vi "SeqLoop.vi"(6 "SEQ STEP Display":refnum<notifier>, 8 "error in (no error)":errorcluster, 9 "SEQ":refnum<queue>, 10 "CORE":refnum<queue>, 11 "WINFAS 2 Data Queue":T3) -> (0 "error out":errorcluster)   [LabVIEW 2014, in "SeqLoop.lvlib"]
uses:
  SeqLoop.lvlib
  APIs/Message Queue/Message Cluster.ctl
  APIs/Data Queue/All Data Queues Cluster.ctl
  APIs/Data Queue/Acquisition Data 1 Sample Cluster.ctl
  APIs/Data Queue/Control Data Cluster.ctl
  APIs/Data Queue/Async Acquisition Data Cluster.ctl
  TypeDefs/STEP Display.ctl
  Mimico Display/TypeDefs/Mimic Data.ctl
  Mimico Display/TypeDefs/BG Image.ctl
  Mimico Display/TypeDefs/mObject.ctl
  TypeDefs/Sequence.ctl
  Classes/STEP/STEP.lvclass
  TypeDefs/LogicParsedExpression.ctl
  TypeDefs/Program.ctl
  TypeDefs/HW InOut MAP.ctl
  TypeDefs/Variables State.ctl
  TypeDefs/STEP State.ctl
  Classes/Measurement/Measurement.lvclass
  Classes/AutoZero/AutoZero.lvclass
  Classes/Measurement wRelev/Measurement wRelev.lvclass
  Classes/Relev/Relev.lvclass
  Classes/Measurement wMaster/Measurement wMaster.lvclass
  Classes/Mastering/Mastering.lvclass
  Classes/Scale Calibration/Scale Calibration.lvclass
  APIs/Message Queue/Enqueue Message (Single).vi
  SEQ Monitoring Global Variables.vi
  APIs/Message Queue/WINFAS 2 Message Queue.lvlib
  APIs/Data Queue/WINFAS 2 Data Queue.lvlib
  Mimico Display/Mimico Display.lvlib
panel:
  in  "Empty Sequence":T1
  in  "Current Sequence":T1
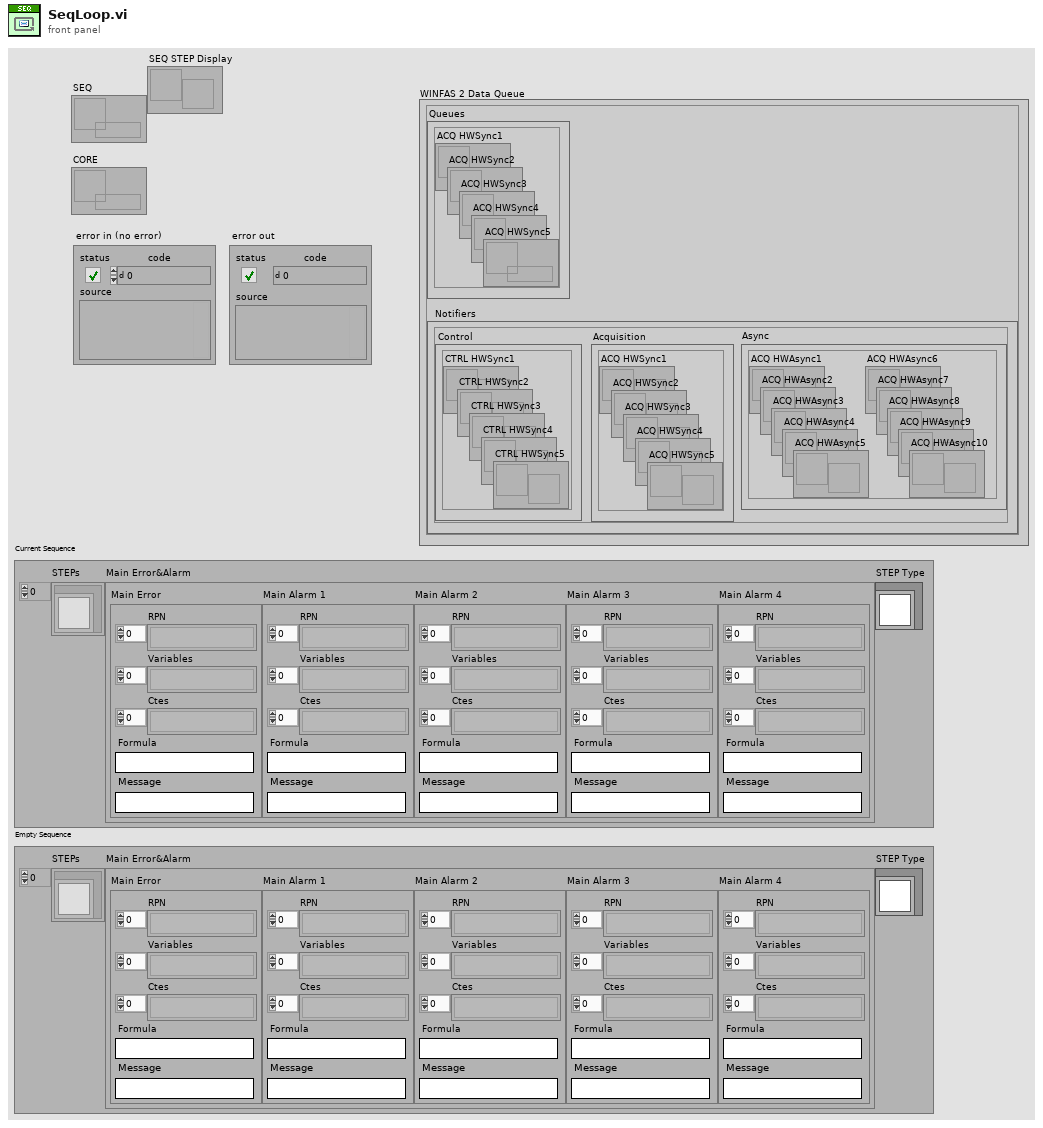
[diagram p1: front panel]
types:
  T1 = typedef "SeqLoop.lvlib/Sequence.ctl" = cluster{"STEPs":refnum<class "STEP.lvclass">[], "Main Error&Alarm":cluster{"Main Error":T2, "Main Alarm 1":T2, "Main Alarm 2":T2, "Main Alarm 3":T2, "Main Alarm 4":T2}, "STEP Type":refnum<class "STEP.lvclass">}
  T2 = typedef "SeqLoop.lvlib/LogicParsedExpression.ctl" = cluster{"RPN ":string[], "Variables":string[], "Ctes":string[], "Formula":string, "Message":string}
  T3 = typedef "WINFAS 2 Data Queue.lvlib/All Data Queues Cluster.ctl" = cluster{"Queues":cluster{"ACQ HWSync1":refnum<queue>, "ACQ HWSync2":refnum<queue>, "ACQ HWSync3":refnum<queue>, "ACQ HWSync4":refnum<queue>, "ACQ HWSync5":refnum<queue>}, "Notifiers":cluster{"Control":cluster{"CTRL HWSync1":refnum<notifier>, "CTRL HWSync2":refnum<notifier>, "CTRL HWSync3":refnum<notifier>, "CTRL HWSync4":refnum<notifier>, "CTRL HWSync5":refnum<notifier>}, "Acquisition":cluster{"ACQ HWSync1":refnum<notifier>, "ACQ HWSync2":refnum<notifier>, "ACQ HWSync3":refnum<notifier>, "ACQ HWSync4":refnum<notifier>, "ACQ HWSync5":refnum<notifier>}, "Async":cluster{"ACQ HWAsync1":refnum<notifier>, "ACQ HWAsync2":refnum<notifier>, "ACQ HWAsync3":refnum<notifier>, "ACQ HWAsync4":refnum<notifier>, "ACQ HWAsync5":refnum<notifier>, "ACQ HWAsync6":refnum<notifier>, "ACQ HWAsync7":refnum<notifier>, "ACQ HWAsync8":refnum<notifier>, "ACQ HWAsync9":refnum<notifier>, "ACQ HWAsync10":refnum<notifier>}}}
  T4 = typedef "SeqLoop.lvlib/STEP State.ctl" = enum16{"Stopped", "First Call", "Idle...", "Advance OK", "Alarm", "Output Security", "Error"}
  T5 = typedef "SeqLoop.lvlib/Variables State.ctl" = cluster{"I":bool[], "P":bool[], "N":bool[], "T":bool[], "X":bool[], "Timer":u32[], "Wait":u32, "Wait?":bool, "Jump":cluster{"Jumping?":bool, "Previous STEP to Jump":u32, "Initial Jump STEP":u32, "STEP Count":u32, "Loop Count":u32, "Number of STEPs":u32, "Repetitions":u32}, "Reset?":bool}
  T6 = typedef "SeqLoop.lvlib/HW InOut MAP.ctl" = cluster{"Inputs":cluster{"Entrada":i32, "Descripción":string, "Habilitada?":bool}[][], "Outputs":cluster{"Salida":i32, "Descripción":string, "Habilitada?":bool, "Formula":string, "Tipo de Salida":string}[][]}
  T7 = typedef "SeqLoop.lvlib/Program.ctl" = cluster{"Prog. Data":cluster{"Tipo de Programa":string, "Operación":i32, "Pieza":i32, "Descripción":string, "Nombre Programa":string, "Autor":string, "Cód. Prog.":i32, "Diseño":string, "Total Meds.:":i32, "Total Meds. Aux.:":i32}, "All Sequences":cluster{"Measurement":T1, "AutoZero":T1, "Special":T1}}
  T8 = cluster{"CTRL HWSync1":refnum<notifier>, "CTRL HWSync2":refnum<notifier>, "CTRL HWSync3":refnum<notifier>, "CTRL HWSync4":refnum<notifier>, "CTRL HWSync5":refnum<notifier>}
  T9 = cluster{"File Direction":path, "Progs Data":variant}
  T10 = cluster{"element":cluster{"File Direction":path, "Progs Data":variant}, "Program Type":string}
  T11 = typedef "SeqLoop.lvlib/HW CTRL Data.ctl" = cluster{"Inputs":bool[], "Encoder 1":sgl, "Encoder 2":sgl, "Encoder 3":sgl, "Encoder 4":sgl, "Encoder 5":sgl}
  T12 = cluster{"Alarm 1":bool, "Alarm 2":bool, "Alarm 3":bool, "Alarm 4":bool, "Main Err&Alarm?":bool}
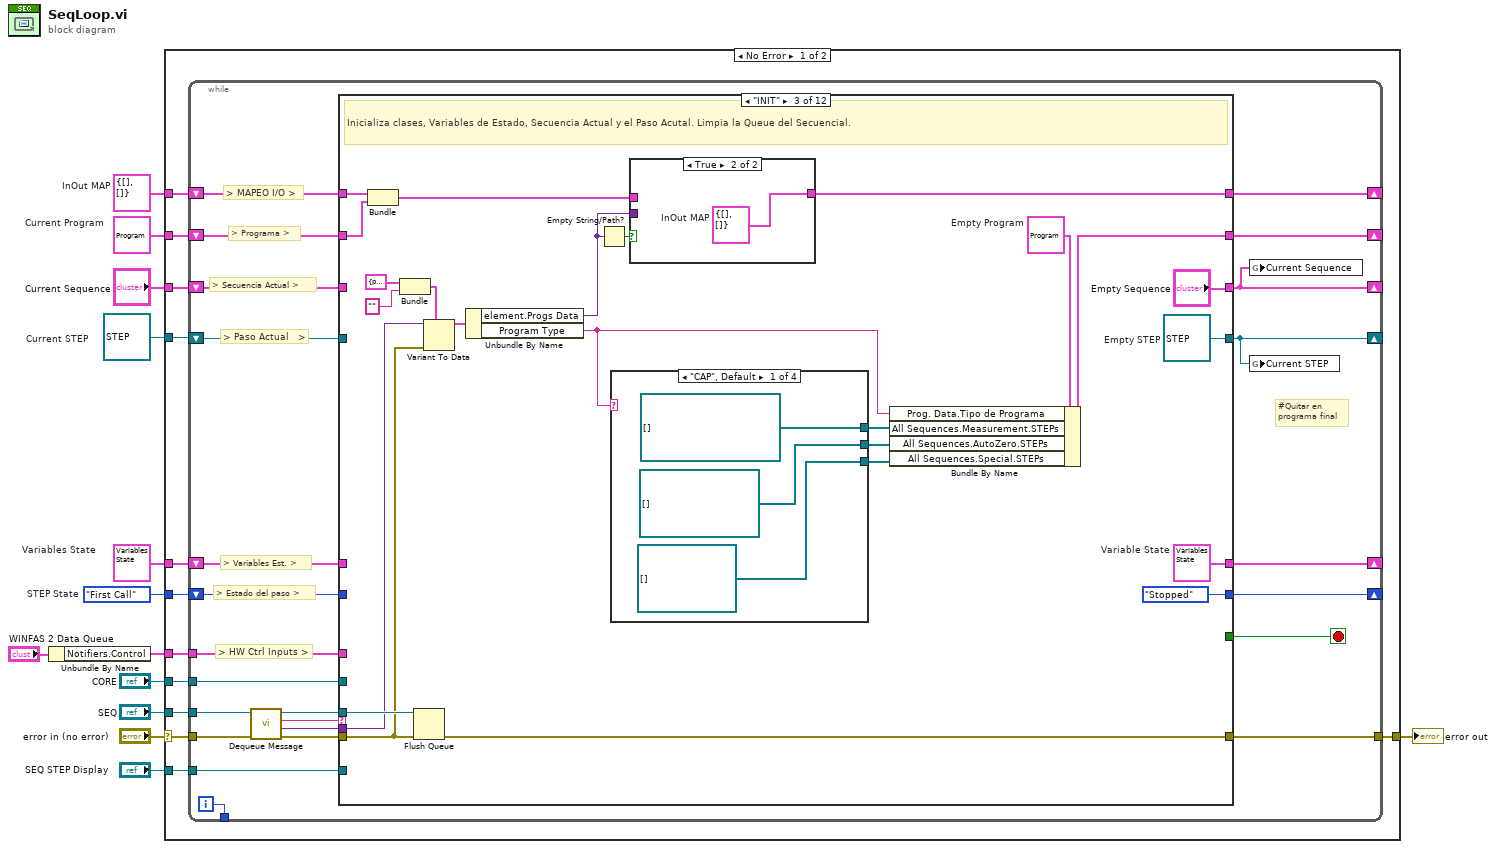
[diagram p0: block diagram]
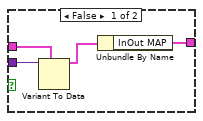
[diagram p4: hidden frame]
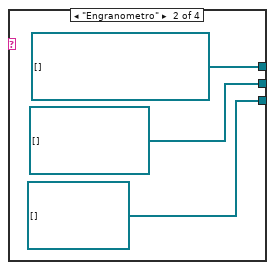
[diagram p5: hidden frame]
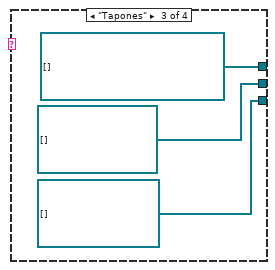
[diagram p6: hidden frame]
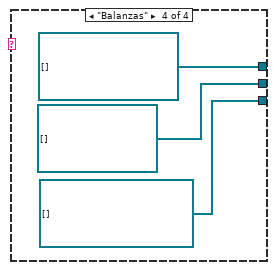
[diagram p7: hidden frame]
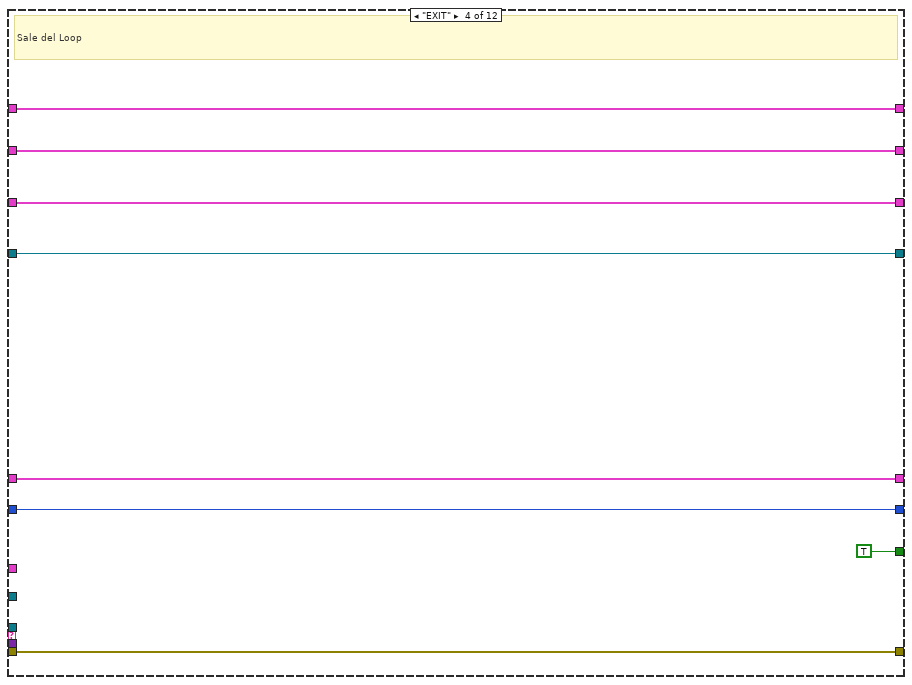
[diagram p8: hidden frame]
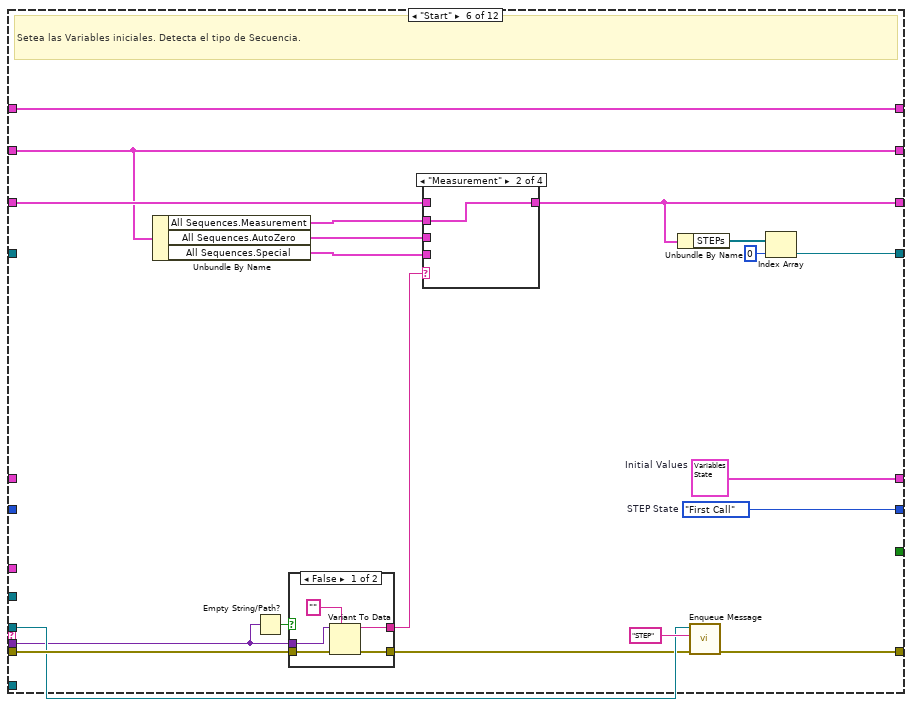
[diagram p10: hidden frame]
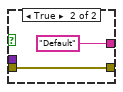
[diagram p11: hidden frame]
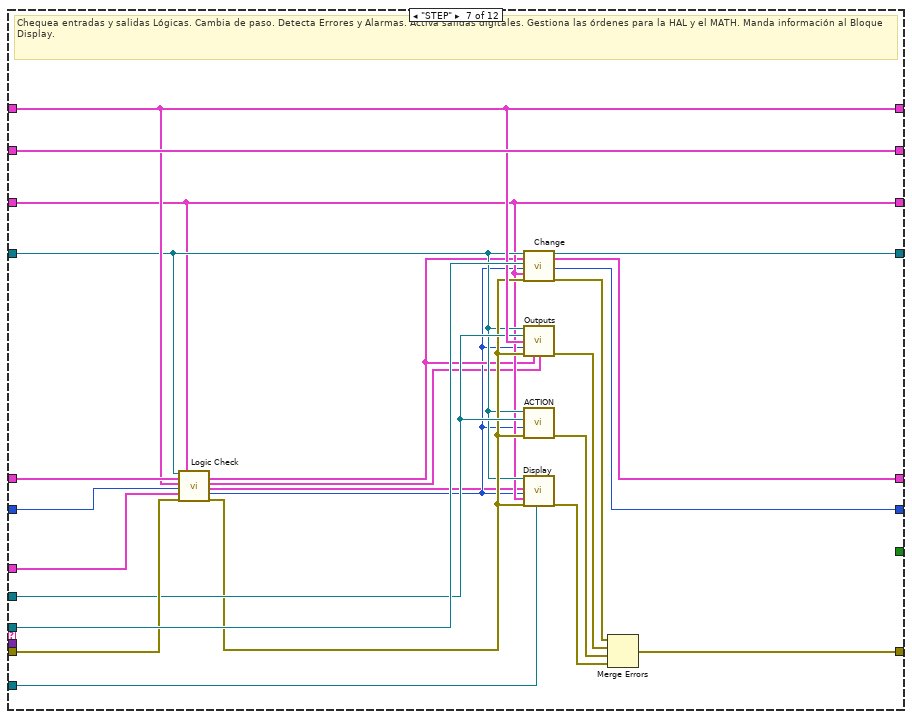
[diagram p15: hidden frame]
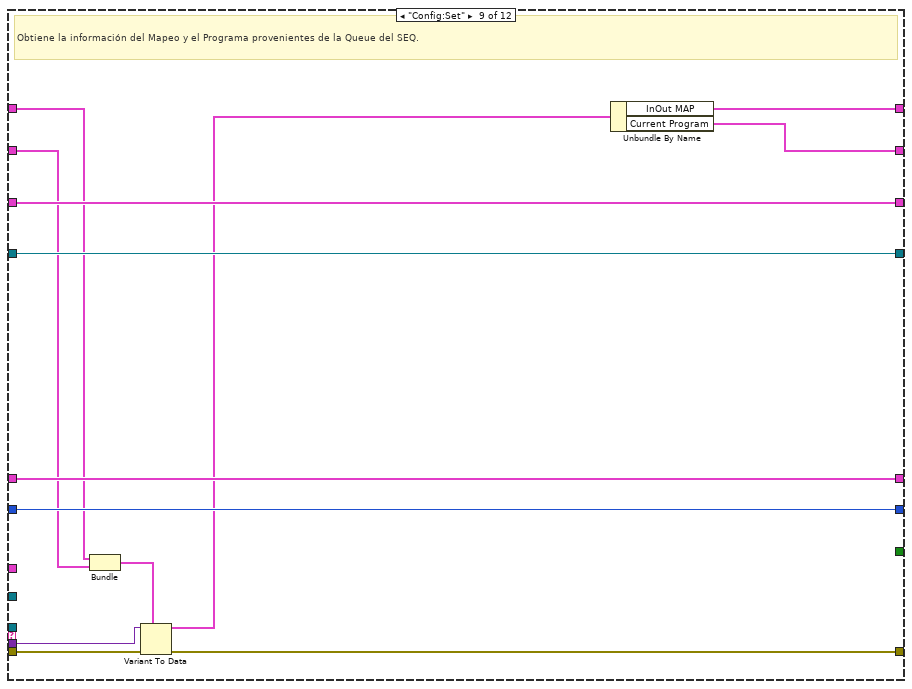
[diagram p17: hidden frame]
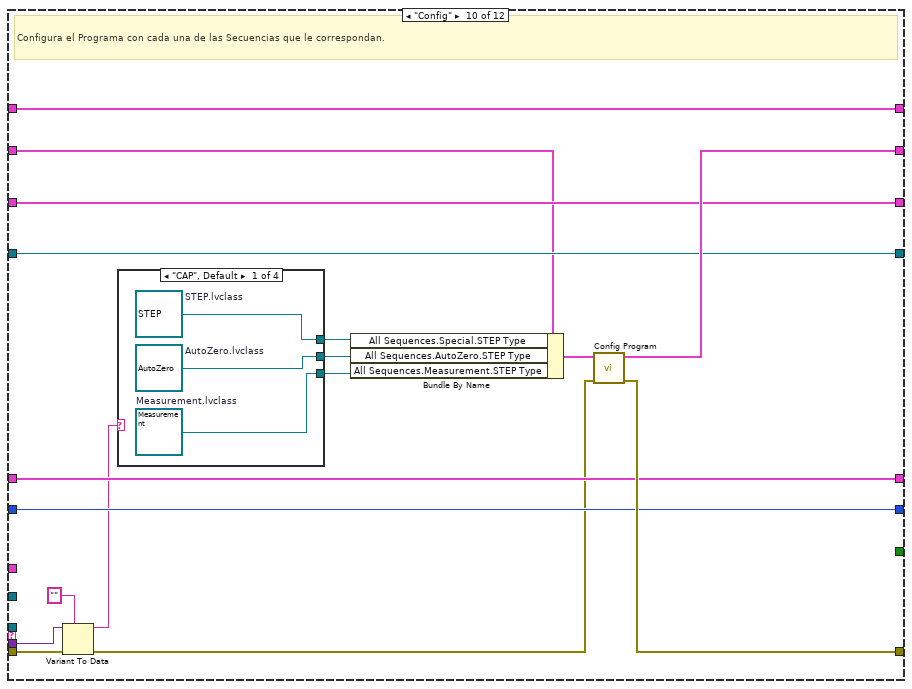
[diagram p18: hidden frame]
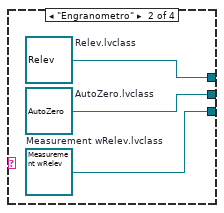
[diagram p19: hidden frame]
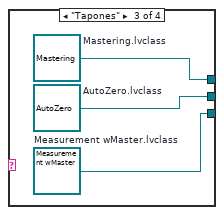
[diagram p20: hidden frame]
diagram:
  w3 = refnum<class "STEP.lvclass"> refnum  # Current STEP
  w6 = STEP_State."First Call"  # STEP State
  w7 = T5 {"I"=[], "P"=[], "N"=[], "T"=[], "X"=[], "Timer"=[], "Wait"=0, "Wait?"=FALSE, "Jump"={"Jumping?"=FALSE, "Previous STEP to Jump"=0, "Initial Jump STEP"=0, "STEP Count"=0, "Loop Count"=0, "Number of STEPs"=0, "Repetitions"=0}, "Reset?"=FALSE}  # Variables State
  w9 = T6 {"Inputs"=[], "Outputs"=[]}  # InOut MAP
  w8 = T7 {"Prog. Data"={"Tipo de Programa"="", "Operación"=0, "Pieza"=0, "Descripción"="", "Nombre Programa"="", "Autor"="", "Cód. Prog."=0, "Diseño"="", "Total Meds.:"=0, "Total Meds. Aux.:"=0}, "All Sequences"={"Measurement"={"STEPs"=[], "Main Error&Alarm"={"Main Error"={"RPN "=[], "Variables"=[], "Ctes"=[], "Formula"="", "Message"=""}, "Main Alarm 1"={"RPN "=[], "Variables"=[], "Ctes"=[], "Formula"="", "Message"=""}, "Main Alarm 2"={"RPN "=[], "Variables"=[], "Ctes"=[], "Formula"="", "Message"=""}, "Main Alarm 3"={"RPN "=[], "Variables"=[], "Ctes"=[], "Formula"="", "Message"=""}, "Main Alarm 4"={"RPN "=[], "Variables"=[], "Ctes"=[], "Formula"="", "Message"=""}}, "STEP Type"=refnum}, "AutoZero"={"STEPs"=[], "Main Error&Alarm"={"Main Error"={"RPN "=[], "Variables"=[], "Ctes"=[], "Formula"="", "Message"=""}, "Main Alarm 1"={"RPN "=[], "Variables"=[], "Ctes"=[], "Formula"="", "Message"=""}, "Main Alarm 2"={"RPN "=[], "Variables"=[], "Ctes"=[], "Formula"="", "Message"=""}, "Main Alarm 3"={"RPN "=[], "Variables"=[], "Ctes"=[], "Formula"="", "Message"=""}, "Main Alarm 4"={"RPN "=[], "Variables"=[], "Ctes"=[], "Formula"="", "Message"=""}}, "STEP Type"=refnum}, "Special"={"STEPs"=[], "Main Error&Alarm"={"Main Error"={"RPN "=[], "Variables"=[], "Ctes"=[], "Formula"="", "Message"=""}, "Main Alarm 1"={"RPN "=[], "Variables"=[], "Ctes"=[], "Formula"="", "Message"=""}, "Main Alarm 2"={"RPN "=[], "Variables"=[], "Ctes"=[], "Formula"="", "Message"=""}, "Main Alarm 3"={"RPN "=[], "Variables"=[], "Ctes"=[], "Formula"="", "Message"=""}, "Main Alarm 4"={"RPN "=[], "Variables"=[], "Ctes"=[], "Formula"="", "Message"=""}}, "STEP Type"=refnum}}}  # Current Program
  n1 = Unbundle By Name("WINFAS 2 Data Queue") -> ("Notifiers.Control"=w4:T8)
  n2 = case shown="No Error" "error in (no error)" {
    selector: "error in (no error)" -> [w25 w245]
    tunnel: [w18 w245] -> w12
    tunnel: "CORE" -> [w24 _]
    tunnel: "SEQ" -> [w23 _]
    tunnel: w9 -> [w22 _]
    tunnel: w8 -> [w21 _]
    tunnel: "Current Sequence" -> [w17 _]
    tunnel: w7 -> [w20 _]
    tunnel: "SEQ STEP Display" -> [w19 _]
    tunnel: w6 -> [w16 _]
    tunnel: w4 -> [w15 _]
    tunnel: w3 -> [w14 _]
    frame No Error {
      n3 = while {
        tunnel: w25 -> [w45]
        tunnel: [w33] -> w18
        tunnel: w23 -> [w46]
        shift-right: [w47] -> _
        shift-left: w20 -> [w48]
        shift-right: [w40] -> _
        shift-left: w22 -> [w41]
        shift-right: [w38] -> _
        shift-left: w21 -> [w39]
        tunnel: w24 -> [w37]
        tunnel: w19 -> [w36]
        shift-right: [w27] -> _
        shift-left: w17 -> [w34]
        tunnel: w15 -> [w35]
        shift-right: [w28] -> _
        shift-left: w14 -> [w30]
        shift-right: [w29] -> _
        shift-left: w16 -> [w31]
        tunnel: [w26] -> _
        i -> [w26]
        stop <- w49 stop-if-true
        # "#Quitar en\nprograma final"
        # "> HW Ctrl Inputs >"
        # "> Variables Est. >"
        # "> Estado del paso >"
        # "> Paso Actual   >"
        # "> Secuencia Actual >"
        # "> Programa >"
        # "> MAPEO I/O >"
        n4 = call "Dequeue Message.vi"("error in (no error)"=w45, "Message Queue"=w46) -> ("error out"=w44:errorcluster, "Message Data"=w42:variant, "Message"=w43:string, "dup Message Queue"=w32:refnum<queue>)  [unwired: 6 in]
        n5 = case shown="\"INIT\"" w43 {
          tunnel: [w55 w59 w85 w110 w119 w131 w168 w180 w183 w211 w232 w241] -> w33
          tunnel: w44 -> [w55 w59 w80 w110 w119 w137 w163 w180 w193 w202 w224 w242]
          tunnel: w42 -> [_ _ w79 _ _ w121 _ _ w192 w195 _ _]
          tunnel: [_ _ _ TRUE _ _ _ _ _ _ _ _] -> w49
          tunnel: w48 -> [w56 w63 _ w111 w118 _ w166 w181 w194 w210 w231 w244]
          tunnel: [w56 w63 w86 w111 w118 w128 w156 w181 w194 w210 w231 w244] -> w47
          tunnel: w41 -> [w52 w61 w69 w107 w116 w135 w162 w177 w186 w209 w230 w235]
          tunnel: [w52 w61 w67 w107 w116 w135 w162 w177 w189 w209 w229 w235] -> w40
          tunnel: w39 -> [w54 w62 w68 w109 w117 w132 w171 w179 w185 w200 w228 w234]
          tunnel: [w54 w62 w81 w109 w117 w132 w171 w179 w190 w208 w228 w234] -> w38
          tunnel: w37 -> [_ _ _ _ _ _ w161 _ _ _ _ w243]
          tunnel: w36 -> [_ _ _ _ _ _ w165 _ _ _ _ _]
          tunnel: [w53 w60 "Empty Sequence" w108 w115 w124 w155 w178 w191 w207 w227 w239] -> w27
          tunnel: w34 -> [w53 w60 _ w108 w115 w133 w155 w178 w191 w207 w227 w239]
          tunnel: w35 -> [_ _ _ _ _ _ w167 _ _ _ _ _]
          tunnel: w32 -> [_ _ w87 _ _ w134 w169 _ _ _ _ _]
          tunnel: w31 -> [w50 w57 _ w105 w113 _ w164 w175 w187 w205 w225 w237]
          tunnel: [w51 w58 w84 w106 w114 w122 w172 w176 w188 w206 w226 w238] -> w28
          tunnel: w30 -> [w51 w58 _ w106 w114 _ w157 w176 w188 w206 w226 w238]
          tunnel: [w50 w57 STEP_State."Stopped" ("STEP State") w105 w113 w126 w170 w175 w187 w205 w225 w237] -> w29
          frame "----LOOP----" {
            # "Bloque que adminte futuras configuraciones al inicio."
          }
          frame Default {
          }
          frame "INIT" {
            w84 = refnum<class "STEP.lvclass"> refnum  # Empty STEP
            w82 = T7 {"Prog. Data"={"Tipo de Programa"="", "Operación"=0, "Pieza"=0, "Descripción"="", "Nombre Programa"="", "Autor"="", "Cód. Prog."=0, "Diseño"="", "Total Meds.:"=0, "Total Meds. Aux.:"=0}, "All Sequences"={"Measurement"={"STEPs"=[], "Main Error&Alarm"={"Main Error"={"RPN "=[], "Variables"=[], "Ctes"=[], "Formula"="", "Message"=""}, "Main Alarm 1"={"RPN "=[], "Variables"=[], "Ctes"=[], "Formula"="", "Message"=""}, "Main Alarm 2"={"RPN "=[], "Variables"=[], "Ctes"=[], "Formula"="", "Message"=""}, "Main Alarm 3"={"RPN "=[], "Variables"=[], "Ctes"=[], "Formula"="", "Message"=""}, "Main Alarm 4"={"RPN "=[], "Variables"=[], "Ctes"=[], "Formula"="", "Message"=""}}, "STEP Type"=refnum}, "AutoZero"={"STEPs"=[], "Main Error&Alarm"={"Main Error"={"RPN "=[], "Variables"=[], "Ctes"=[], "Formula"="", "Message"=""}, "Main Alarm 1"={"RPN "=[], "Variables"=[], "Ctes"=[], "Formula"="", "Message"=""}, "Main Alarm 2"={"RPN "=[], "Variables"=[], "Ctes"=[], "Formula"="", "Message"=""}, "Main Alarm 3"={"RPN "=[], "Variables"=[], "Ctes"=[], "Formula"="", "Message"=""}, "Main Alarm 4"={"RPN "=[], "Variables"=[], "Ctes"=[], "Formula"="", "Message"=""}}, "STEP Type"=refnum}, "Special"={"STEPs"=[], "Main Error&Alarm"={"Main Error"={"RPN "=[], "Variables"=[], "Ctes"=[], "Formula"="", "Message"=""}, "Main Alarm 1"={"RPN "=[], "Variables"=[], "Ctes"=[], "Formula"="", "Message"=""}, "Main Alarm 2"={"RPN "=[], "Variables"=[], "Ctes"=[], "Formula"="", "Message"=""}, "Main Alarm 3"={"RPN "=[], "Variables"=[], "Ctes"=[], "Formula"="", "Message"=""}, "Main Alarm 4"={"RPN "=[], "Variables"=[], "Ctes"=[], "Formula"="", "Message"=""}}, "STEP Type"=refnum}}}  # Empty Program
            w86 = T5 {"I"=[], "P"=[], "N"=[], "T"=[], "X"=[], "Timer"=[], "Wait"=0, "Wait?"=FALSE, "Jump"={"Jumping?"=FALSE, "Previous STEP to Jump"=0, "Initial Jump STEP"=0, "STEP Count"=0, "Loop Count"=0, "Number of STEPs"=0, "Repetitions"=0}, "Reset?"=FALSE}  # Variable State
            # "Inicializa clases, Variables de Estado, Secuencia Actual y el Paso Acutal. Limpia la Queue del Secuencial."
            n6 = Bundle("InOut MAP"=w69, "Current Program"=w68) -> (w70:cluster{"InOut MAP":T6, "Current Program":T7})  [unwired: 1 in]
            n7 = Bundle("element"=T9 {"File Direction"=path "", "Progs Data"=variant}, "Program Type"="") -> (w71:T10)  [unwired: 1 in]
            n8 = Flush Queue(queue=w87, error in (no error)=w80) -> (error out=w85:errorcluster)  [unwired: 2 out]
            n9 = Variant To Data(error in=w80, type=w71, Variant=w79) -> (data=w74:T10)  [unwired: 1 out]
            n10 = Unbundle By Name(w74) -> ("element.Progs Data"=w66:variant, "Program Type"=w64:string)
            n11 = Empty String/Path?(string/path=w66) -> (empty?=w65:bool)
            n12 = case shown="\"CAP\", Default" w64 {
              tunnel: [refnum<class "Measurement.lvclass">[] [] refnum<class "Measurement wRelev.lvclass">[] [] refnum<class "Measurement wMaster.lvclass">[] [] refnum<class "Measurement.lvclass">[] []] -> w78
              tunnel: [refnum<class "AutoZero.lvclass">[] [] refnum<class "AutoZero.lvclass">[] [] refnum<class "AutoZero.lvclass">[] [] refnum<class "AutoZero.lvclass">[] []] -> w77
              tunnel: [refnum<class "STEP.lvclass">[] [] refnum<class "Relev.lvclass">[] [] refnum<class "Mastering.lvclass">[] [] refnum<class "Scale Calibration.lvclass">[] []] -> w76
              frame "CAP", Default {
              }
              frame "Engranometro" {
              }
              frame "Tapones" {
              }
              frame "Balanzas" {
              }
            }
            n13 = case shown="True" w65 {
              tunnel: w70 -> [w91 _]
              tunnel: [w89 w92] -> w67
              tunnel: w66 -> [w88 _]
              frame False {
                n14 = Variant To Data(type=w91, Variant=w88) -> (data=w90:cluster{"InOut MAP":T6, "Current Program":T7})  [unwired: 1 in, 1 out]
                n15 = Unbundle By Name(w90) -> ("InOut MAP"=w89:T6)
              }
              frame True {
                w92 = T6 {"Inputs"=[], "Outputs"=[]}  # InOut MAP
              }
            }
            n16 = Bundle By Name(cluster=w82, "Prog. Data.Tipo de Programa"=w64, "All Sequences.Measurement.STEPs"=w78, "All Sequences.AutoZero.STEPs"=w77, "All Sequences.Special.STEPs"=w76) -> (w81:T7)
          }
          frame "EXIT" {
            # "Sale del Loop"
          }
          frame "----ACTION----" {
          }
          frame "Start" {
            w126 = STEP_State."First Call"  # STEP State
            w128 = T5 {"I"=[], "P"=[], "N"=[], "T"=[], "X"=[], "Timer"=[], "Wait"=0, "Wait?"=FALSE, "Jump"={"Jumping?"=FALSE, "Previous STEP to Jump"=0, "Initial Jump STEP"=0, "STEP Count"=0, "Loop Count"=0, "Number of STEPs"=0, "Repetitions"=0}, "Reset?"=FALSE}  # Initial Values
            # "Setea las Variables iniciales. Detecta el tipo de Secuencia."
            n17 = Unbundle By Name(w132) -> ("All Sequences.Measurement"=w139:T1, "All Sequences.AutoZero"=w138:T1, "All Sequences.Special"=w129:T1)
            n18 = Empty String/Path?(string/path=w121) -> (empty?=w120:bool)
            n19 = case shown="False" w120 {
              tunnel: w137 -> [w144 w146]
              tunnel: [w142 "Default"] -> w130
              tunnel: [w141 w146] -> w125
              tunnel: w121 -> [w140 _]
              frame False {
                n20 = Variant To Data(error in=w144, type="", Variant=w140) -> (data=w142:string, error out=w141:errorcluster)
              }
              frame True {
              }
            }
            n21 = case shown="\"Measurement\"" w130 {
              tunnel: w139 -> [_ w148 _ _]
              tunnel: w138 -> [_ _ w149 _]
              tunnel: [w147 w148 w149 w150] -> w124
              tunnel: w133 -> [w147 _ _ _]
              tunnel: w129 -> [_ _ _ w150]
              frame Default {
              }
              frame "Measurement" {
              }
              frame "Auto-Zero" {
              }
              frame "Special" {
              }
            }
            n22 = Unbundle By Name(w124) -> ("STEPs"=w123:refnum<class "STEP.lvclass">[])
            n23 = call-poly "Enqueue Message.vi"("error in (no error)"=w125, "Message"="STEP", "Message Queue"=w134) -> ("error out"=w131:errorcluster)  [unwired: 7 in, 1 out]
            n24 = Index Array(array=w123, index=0) -> (element=w122:refnum<class "STEP.lvclass">)
          }
          frame "STEP" {
            # "Chequea entradas y salidas Lógicas. Cambia de paso. Detecta Errores y Alarmas. Activa salidas digitales. Gestiona las órdenes para la HAL y el MATH. Manda información al Bloque Display."
            n25 = call "Logic Check.vi"("STEP in"=w157, "Variables State in"=w166, "HW InOut MAP"=w162, "STEP State in"=w164, "Notifiers.Control"=w167, "error in (no error)"=w163, "Current Sequence"=w155) -> ("Variables State out"=w154:T5, "HW CTRL Data"=w151:T11, "Alarms triggered?"=w152:T12, "STEP State out"=w153:T4, "error out"=w160:errorcluster)  [unwired: 7 in, 1 out]
            n26 = call "Change.vi"("STEP in"=w157, "Variables State"=w154, "SEQ"=w169, "STEP State"=w153, "Current Sequence"=w155, "error in (no error)"=w160) -> ("STEP out"=w172:refnum<class "STEP.lvclass">, "Variables State out"=w156:T5, "STEP State out"=w170:T4, "error out"=w159:errorcluster)  [unwired: 10 in]
            n27 = call "Outputs.vi"("STEP in"=w157, "CORE"=w161, "Mapping Buss"=w162, "STEP State"=w153, "error in (no error)"=w160, "Variables State in"=w154, "HW CTRL Data"=w151) -> ("error out"=w158:errorcluster)  [unwired: 7 in, 1 out]
            n28 = call-dynamic "ACTION.vi"("error in (no error)"=w160, "STEP State"=w153, "CORE"=w161, "STEP in"=w157) -> ("error out"=w174:errorcluster)  [unwired: 6 in, 1 out]
            n29 = call "Display.vi"("STEP in"=w157, "Alarms triggered?"=w152, "STEP State"=w153, "Current Sequence"=w155, "error in (no error)"=w160, "SEQ STEP Display"=w165) -> ("error out"=w173:errorcluster)  [unwired: 12 in, 1 out]
            n30 = Merge Errors(w159, w158, w174, w173) -> (w168:errorcluster)
          }
          frame "----UTILITY----" {
          }
          frame "Config:Set" {
            # "Obtiene la información del Mapeo y el Programa provenientes de la Queue del SEQ."
            n31 = Bundle("InOut MAP"=w186, "Current Program"=w185) -> (w184:cluster{"InOut MAP":T6, "Current Program":T7})  [unwired: 1 in]
            n32 = Variant To Data(error in=w193, type=w184, Variant=w192) -> (data=w182:cluster{"InOut MAP":T6, "Current Program":T7}, error out=w183:errorcluster)
            n33 = Unbundle By Name(w182) -> ("InOut MAP"=w189:T6, "Current Program"=w190:T7)
          }
          frame "Config" {
            # "Configura el Programa con cada una de las Secuencias que le correspondan."
            n34 = Variant To Data(error in=w202, type="", Variant=w195) -> (data=w204:string, error out=w201:errorcluster)
            n35 = case shown="\"CAP\", Default" w204 {
              tunnel: [w214 w216 w219 w223] -> w198
              tunnel: [w213 w217 w220 w222] -> w197
              tunnel: [w212 w215 w218 w221] -> w196
              frame "CAP", Default {
                w212 = refnum<class "STEP.lvclass"> refnum  # STEP.lvclass
                w213 = refnum<class "AutoZero.lvclass"> refnum  # AutoZero.lvclass
                w214 = refnum<class "Measurement.lvclass"> refnum  # Measurement.lvclass
              }
              frame "Engranometro" {
                w215 = refnum<class "Relev.lvclass"> refnum  # Relev.lvclass
                w217 = refnum<class "AutoZero.lvclass"> refnum  # AutoZero.lvclass
                w216 = refnum<class "Measurement wRelev.lvclass"> refnum  # Measurement wRelev.lvclass
              }
              frame "Tapones" {
                w218 = refnum<class "Mastering.lvclass"> refnum  # Mastering.lvclass
                w220 = refnum<class "AutoZero.lvclass"> refnum  # AutoZero.lvclass
                w219 = refnum<class "Measurement wMaster.lvclass"> refnum  # Measurement wMaster.lvclass
              }
              frame "Balanzas" {
                w221 = refnum<class "Scale Calibration.lvclass"> refnum  # Scale Calibration.lvclass
                w222 = refnum<class "AutoZero.lvclass"> refnum  # AutoZero.lvclass
                w223 = refnum<class "Measurement.lvclass"> refnum  # Measurement.lvclass
              }
            }
            n36 = Bundle By Name(cluster=w200, "All Sequences.Special.STEP Type"=w196, "All Sequences.AutoZero.STEP Type"=w197, "All Sequences.Measurement.STEP Type"=w198) -> (w199:T7)
            n37 = call "Config Program.vi"("error in (no error)"=w201, "Prog in"=w199) -> ("error out"=w211:errorcluster, "Prog out"=w208:T7)  [unwired: 8 in]
          }
          frame "Config:IO" {
            # "Configura el Mapeo correspondiente al Programa utilizado."
            n38 = call "Config Mapping.vi"("error in (no error)"=w224, "HW InOut MAP in"=w230) -> ("error out"=w232:errorcluster, "HW InOut MAP out"=w229:T6)  [unwired: 8 in]
          }
          frame "Config:Get" {
            # "Envia la informacion del Mapeo y dal Programa al CORE para ser procesados posteriormente."
            n39 = Bundle("InOut MAP"=w235, "Current Program"=w234) -> (w233:cluster{"InOut MAP":T6, "Current Program":T7})  [unwired: 1 in]
            n40 = To Variant(anything=w233) -> (Variant=w236:variant)
            n41 = call-poly "Enqueue Message.vi"("error in (no error)"=w242, "Message Data"=w236, "Message"="CONFIG", "Message Queue"=w243) -> ("error out"=w241:errorcluster)  [unwired: 6 in, 1 out]
          }
        }
        n42 = global write "SEQ Monitoring Global Variables.vi" "Current Sequence"(w27) -> ()
        n43 = global write "SEQ Monitoring Global Variables.vi" "Current STEP"(w28) -> ()
      }
    }
    frame Error {
    }
  }
  "error out" <- w12
